vi "calc robot plan graph.vi"(6 "2x scale":bool, 11 "pitch":dbl) -> (1 "Angle (in)":dbl[](array[numeric])=[nan, nan], 2 "XY Graph values":cluster{"X Out":dbl[], "Y Out":dbl[]}[](array[cluster]), 3 "Stroke (in)":dbl[](array[numeric])=[nan, nan])   [LabVIEW 2020]
uses:
  <vilib>/Analysis/coordinate.llb/2D Cartesian Coordinate Rotation (Array).vi
  Robot Global Data.vi
  <vilib>/Rock Robotics/Network Tables/NT Read Number.vi
  <vilib>/Analysis/NI_AALPro.lvlib
panel:
  out "Diff in shoulder Y":dbl
  in  "TESTING?":bool
  out "arctan(x)":dbl
  out "x/y":dbl
  in  "shoulder width":dbl
  out "climber (in)":dbl[](array[numeric])
  out "hook @ retracted":dbl[](array[numeric])
  out "convert arm inches to degrees":dbl
  out "convert arm inches to revs":dbl
  out "convert climber inches to tics":dbl
  out "read pos revs":dbl[](array[numeric])
  out "read climber tics":dbl[](array[numeric])
  out "Ybars":dbl[](array[numeric])
  out "Y hi bar":dbl
  out "Y mid bar":dbl
  out "Yshoulder":dbl[](array[numeric]) format="%#_5g"
  out "Lsin()":dbl[](array[numeric]) format="%#_4f"
  out "Lcos()":dbl[](array[numeric]) format="%#.4f"
  out "arm length (in)":dbl[](array[numeric])
  out "theta (deg)":dbl[](array[numeric])
  out "arm angle (deg)":dbl[](array[numeric])
  out "HANGAR BARS":T1={"LOW BAR AG"=48.75, "MID BAR AG"=60.25, "HIGH BAR AG"=75.625, "TRAV BAR AG"=91.0, "BAR OD"=1.66, "SPACING"=24.0}
  in  "graph height":dbl=48.0
  in  "graph width":dbl=48.0
  in  "robot frame length":dbl=29.5
  in  "robot frame width":dbl=30.0
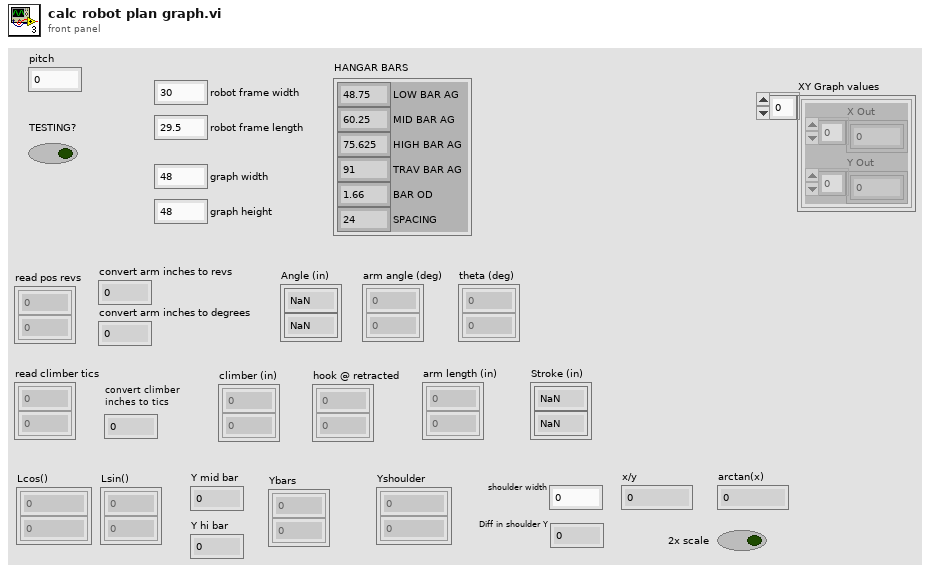
[diagram p1: front panel]
types:
  T1 = cluster{"LOW BAR AG":dbl, "MID BAR AG":dbl, "HIGH BAR AG":dbl, "TRAV BAR AG":dbl, "BAR OD":dbl, "SPACING":dbl}
  T2 = cluster{"MIN":dbl, "MAX":dbl, "convert climber inches to tics":dbl, "INITIALIZE":dbl}
  T3 = cluster{"MIN":dbl, "MAX":dbl, "convert arm inches to revs":dbl, "convert arm inches to degrees":dbl}
  T4 = cluster{"HOOK CTR LENGTH LEFT":dbl, "HOOK CTR LENGTH RIGHT":dbl, "HOOK DEPTH":dbl, "HOOK ID":dbl, "SHOULDER PIN AG":dbl, "ARM DIFF RT-LEFT":dbl}
  T5 = cluster{"gear ratio":cluster{"value":dbl, "descr":string}, "screw tpi":cluster{"value":dbl, "descr":string}, "shoulder AG":cluster{"value":dbl, "descr":string}, "shoulder to CTR":cluster{"value":dbl, "descr":string}, "shoulder to screw 0":cluster{"value":dbl, "descr":string}, "screw shuttle AG":cluster{"value":dbl, "descr":string}, "screw length":cluster{"value":dbl, "descr":string}, "screw to full front":cluster{"value":dbl, "descr":string}, "screw link":cluster{"value":dbl, "descr":string}, "lower arm length":cluster{"value":dbl, "descr":string}, "arm top":cluster{"value":dbl, "descr":string}, "shoulder to pin link Y":cluster{"value":dbl, "descr":string}, "shoulder to pin link X":cluster{"value":dbl, "descr":string}, "hook ht":cluster{"value":dbl, "descr":string}, "hook clear":cluster{"value":dbl, "descr":string}}
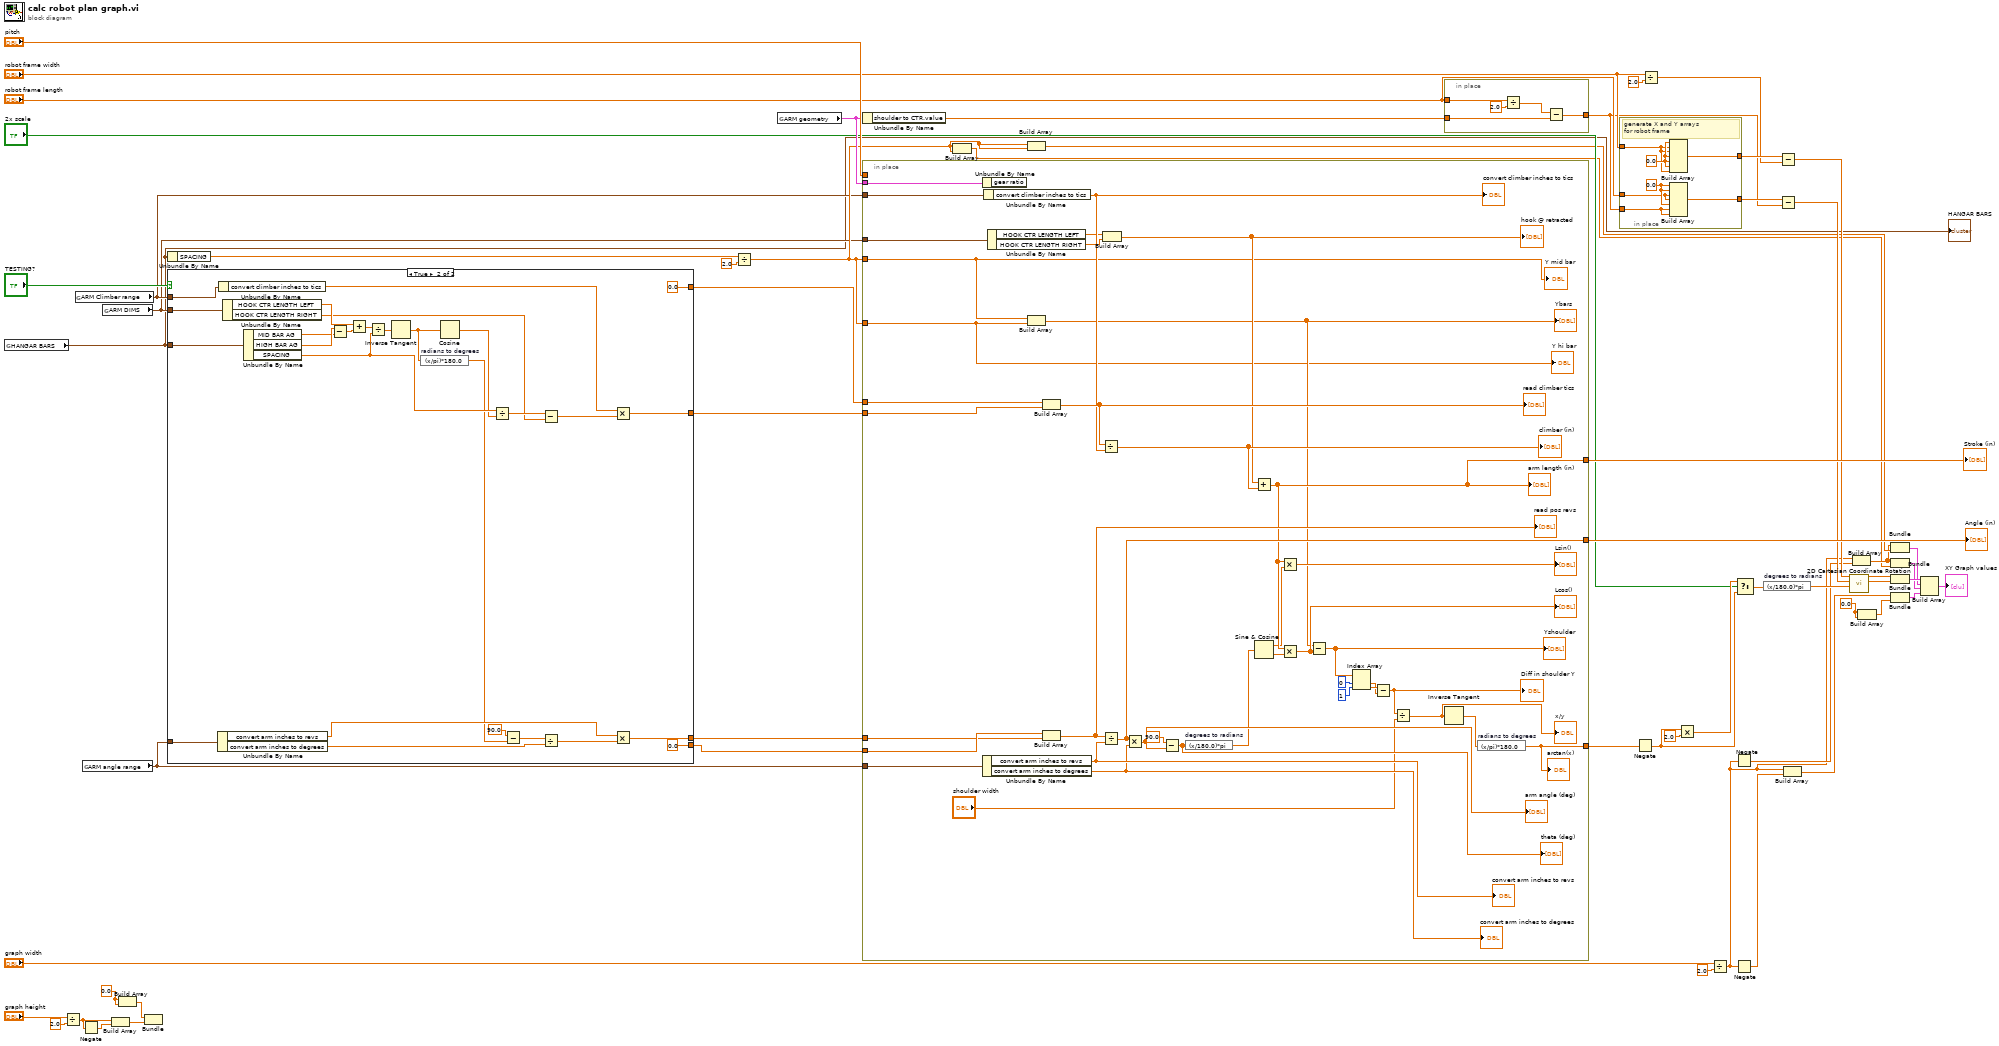
[diagram p0: block diagram]
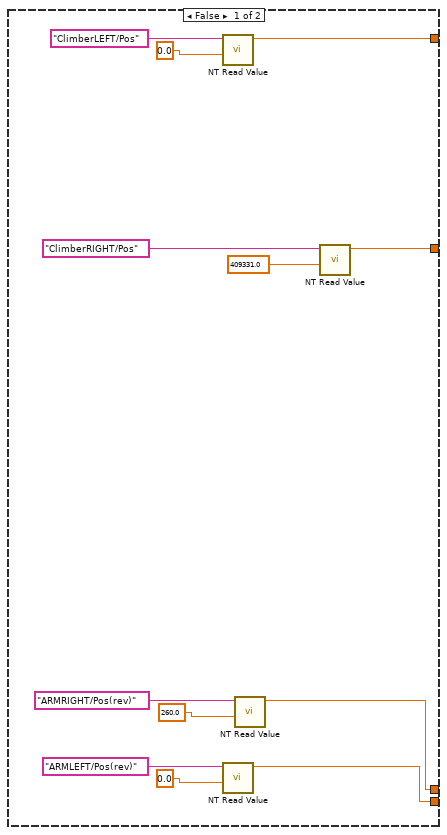
[diagram p2: hidden frame]
diagram:
  w13 = 0.0 ("element")
  w18 = 0.0 ("element")
  n1 = global read "Robot Global Data.vi" "HANGAR BARS"() -> (w1:T1)
  "HANGAR BARS" <- w1
  n2 = Divide(x="graph height", y=2.0) -> (x/y=w17:dbl)
  n3 = global read "Robot Global Data.vi" "ARM Climber range"() -> (w4:T2)
  n4 = global read "Robot Global Data.vi" "ARM angle range"() -> (w2:T3)
  n5 = Negate(x=w17) -> (-x=w16:dbl)
  n6 = global read "Robot Global Data.vi" "ARM DIMS"() -> (w3:T4)
  n7 = Build Array(w17, w16) -> (w22:dbl[])
  n8 = Build Array(w18, w18) -> (w24:dbl[])
  n9 = Bundle(w24, w22) -> ()  [unwired: 1 in, 1 out]
  n10 = Unbundle By Name(w1) -> ("SPACING"=w31:dbl)
  n11 = case shown="True" "TESTING?" {
    tunnel: [w68 0.0 ("Numeric")] -> w9
    tunnel: [w67 w85] -> w8
    tunnel: [w64 0.0 ("Numeric")] -> w7
    tunnel: [w63 w73] -> w6
    tunnel: w4 -> [_ w76]
    tunnel: w3 -> [_ w95]
    tunnel: w2 -> [_ w87]
    tunnel: w1 -> [_ w93]
    frame False {
      n12 = call-poly <vilib>:"NT Read Value.vi"("Default Value"=0.0, "Name"="ClimberLEFT/Pos") -> ("Numeric"=w64:dbl)  [unwired: 8 in, 1 out]
      n13 = call-poly <vilib>:"NT Read Value.vi"("Default Value"=0.0, "Name"="ARMLEFT/Pos(rev)") -> ("Numeric"=w68:dbl)  [unwired: 8 in, 1 out]
      n14 = call-poly <vilib>:"NT Read Value.vi"("Default Value"=260.0, "Name"="ARMRIGHT/Pos(rev)") -> ("Numeric"=w67:dbl)  [unwired: 8 in, 1 out]
      n15 = call-poly <vilib>:"NT Read Value.vi"("Default Value"=409331.0, "Name"="ClimberRIGHT/Pos") -> ("Numeric"=w63:dbl)  [unwired: 8 in, 1 out]
    }
    frame True {
      n16 = Unbundle By Name(w87) -> ("convert arm inches to revs"=w83:dbl, "convert arm inches to degrees"=w86:dbl)
      n17 = Unbundle By Name(w76) -> ("convert climber inches to tics"=w74:dbl)
      n18 = Unbundle By Name(w95) -> ("HOOK CTR LENGTH LEFT"=w92:dbl, "HOOK CTR LENGTH RIGHT"=w77:dbl)
      n19 = Unbundle By Name(w93) -> ("MID BAR AG"=w90:dbl, "HIGH BAR AG"=w91:dbl, "SPACING"=w82:dbl)
      n20 = Subtract(x=w91, y=w90) -> (x-y=w89:dbl)
      n21 = Add(x=w92, y=w89) -> (x+y=w88:dbl)
      n22 = Divide(x=w88, y=w82) -> (x/y=w94:dbl)
      n23 = Inverse Tangent(1:w94) -> (0:w80:dbl)
      n24 = expression code="(x/pi)*180.0" "radians to degrees"(w80) -> (w72:dbl)
      n25 = Cosine(x=w80) -> (cos(x)=w79:dbl)
      n26 = Divide(x=w82, y=w79) -> (x/y=w78:dbl)
      n27 = Subtract(x=90.0, y=w72) -> (x-y=w81:dbl)
      n28 = Subtract(x=w78, y=w77) -> (x-y=w75:dbl)
      n29 = Divide(x=w81, y=w86) -> (x/y=w84:dbl)
      n30 = Multiply(x=w74, y=w75) -> (x*y=w73:dbl)
      n31 = Multiply(x=w83, y=w84) -> (x*y=w85:dbl)
    }
  }
  n32 = Divide(x=w31, y=2.0) -> (x/y=w26:dbl)
  n33 = global read "Robot Global Data.vi" "ARM geometry"() -> (w47:T5)
  n34 = Unbundle By Name(w47) -> ("shoulder to CTR.value"=w52:dbl)
  n35 = in-place {
    in-place-border: w2 -> [w137]
    in-place-border: [w128] -> w56
    in-place-border: w4 -> [w133]
    in-place-border: [w117] -> w57
    in-place-border: w47 -> [w131]
    in-place-border: w3 -> [w130]
    in-place-border: "pitch" -> [_]
    in-place-border: w26 -> [w113]
    in-place-border: w26 -> [w112]
    in-place-border: [w102] -> w41
    in-place-border: w9 -> [w101]
    in-place-border: w8 -> [w100]
    in-place-border: w7 -> [w99]
    in-place-border: w6 -> [w98]
    n36 = Unbundle By Name(w131) -> ()  [unwired: 1 out]
    n37 = Unbundle By Name(w137) -> ("convert arm inches to revs"=w135:dbl, "convert arm inches to degrees"=w129:dbl)
    "convert arm inches to revs" <- w135
    "convert arm inches to degrees" <- w129
    n38 = Unbundle By Name(w133) -> ("convert climber inches to tics"=w132:dbl)
    "convert climber inches to tics" <- w132
    n39 = Unbundle By Name(w130) -> ("HOOK CTR LENGTH LEFT"=w124:dbl, "HOOK CTR LENGTH RIGHT"=w123:dbl)
    n40 = Build Array(w112, w113) -> (w114:dbl[])
    "Ybars" <- w114
    n41 = Build Array(w99, w98) -> (w134:dbl[])
    "read climber tics" <- w134
    n42 = Build Array(w101, w100) -> (w136:dbl[])
    "read pos revs" <- w136
    n43 = Divide(x=w134, y=w132) -> (x/y=w125:dbl[])
    "climber (in)" <- w125
    n44 = Divide(x=w136, y=w135) -> (x/y=w128:dbl[])
    n45 = Build Array(w124, w123) -> (w122:dbl[])
    "hook @ retracted" <- w122
    n46 = Multiply(x=w128, y=w129) -> (x*y=w126:dbl[])
    "arm angle (deg)" <- w126
    n47 = Subtract(x=90.0, y=w126) -> (x-y=w121:dbl[])
    "theta (deg)" <- w121
    n48 = expression code="(x/180.0)*pi" "degrees to radians"(w121) -> (w120:dbl[])
    n49 = Add(x=w122, y=w125) -> (x+y=w117:dbl[])
    "arm length (in)" <- w117
    n50 = Sine & Cosine(0:w120) -> (1:w116:dbl[], 2:w119:dbl[])
    n51 = Multiply(x=w117, y=w116) -> (x*y=→"Lsin()":dbl[])
    n52 = Multiply(x=w117, y=w119) -> (x*y=w115:dbl[])
    "Lcos()" <- w115
    n53 = Subtract(x=w114, y=w115) -> (x-y=w111:dbl[])
    "Yshoulder" <- w111
    n54 = Index Array(array=w111, index #1=0 ("index"), index #2=1 ("index")) -> (element #1=w109:dbl, element #2=w110:dbl)
    n55 = Subtract(x=w110, y=w109) -> (x-y=w106:dbl)
    "Diff in shoulder Y" <- w106
    n56 = Divide(x=w106, y="shoulder width") -> (x/y=w105:dbl)
    "x/y" <- w105
    n57 = Inverse Tangent(1:w105) -> (0:w104:dbl)
    n58 = expression code="(x/pi)*180.0" "radians to degrees"(w104) -> (w102:dbl)
    "arctan(x)" <- w102
    "Y mid bar" <- w112
    "Y hi bar" <- w113
  }
  "Stroke (in)" <- w57
  "Angle (in)" <- w56
  n59 = Build Array(w26, w26) -> (w27:dbl[])
  n60 = Build Array(w26, w26) -> (w29:dbl[])
  n61 = in-place {
    in-place-border: w52 -> [w140]
    in-place-border: "robot frame length" -> [w139]
    in-place-border: [w138] -> w48
    n62 = Divide(x=w139, y=2.0) -> (x/y=w141:dbl)
    n63 = Subtract(x=w141, y=w140) -> (x-y=w138:dbl)
  }
  n64 = in-place {
    in-place-border: "robot frame length" -> [w146]
    in-place-border: "robot frame width" -> [w144]
    in-place-border: [w149] -> w55
    in-place-border: [w148] -> w49
    in-place-border: w48 -> [w143]
    w147 = 0.0 ("element")
    w145 = 0.0 ("element")
    # "generate X and Y arrays\nfor robot frame"
    n65 = Build Array(w145, w144, w144, w145, w145, w145, w144) -> (w149:dbl[])
    n66 = Build Array(w147, w147, w146, w146, w147, w143, w143) -> (w148:dbl[])
  }
  n67 = Negate(x=w41) -> (-x=w43:dbl)
  n68 = Divide(x="robot frame width", y=2.0) -> (x/y=w53:dbl)
  n69 = Multiply(x=w43, y=2.0) -> (x*y=w44:dbl)
  n70 = Divide(x="graph width", y=2.0) -> (x/y=w11:dbl)
  n71 = Negate(x=w11) -> (-x=w19:dbl)
  n72 = Negate(x=w11) -> (-x=w10:dbl)
  n73 = Select(t=w44, s="2x scale", f=w43) -> (s? t:f=w45:dbl)
  n74 = expression code="(x/180.0)*pi" "degrees to radians"(w45) -> (w39:dbl)
  n75 = Subtract(x=w55, y=w53) -> (x-y=w40:dbl[])
  n76 = Subtract(x=w49, y=w48) -> (x-y=w38:dbl[])
  n77 = Build Array(w11, w10) -> (w12:dbl[])
  n78 = call-poly <vilib>:"2D Cartesian Coordinate Rotation.vi"("theta"=w39, "Y"=w38, "X"=w40) -> ("Y Out"=w36:dbl[], "X Out"=w37:dbl[])  [unwired: 6 in, 1 out]
  n79 = Build Array(w11, w19) -> (w28:dbl[])
  n80 = Build Array(w13, w13) -> (w14:dbl[])
  n81 = Bundle(w28, w29) -> (w34:cluster{dbl[], dbl[]})  [unwired: 1 in]
  n82 = Bundle(w28, w27) -> (w33:cluster{dbl[], dbl[]})  [unwired: 1 in]
  n83 = Bundle("X Out"=w37, "Y Out"=w36) -> (w35:cluster{"X Out":dbl[], "Y Out":dbl[]})  [unwired: 1 in]
  n84 = Bundle(w12, w14) -> (w15:cluster{dbl[], dbl[]})  [unwired: 1 in]
  n85 = Build Array(w35, w34, w33, w15) -> (→"XY Graph values":cluster{"X Out":dbl[], "Y Out":dbl[]}[])
